vi "Resolve Actions.vi"(7 "Round":u32, 9 "Teams in":refnum<class "Team.lvclass">[](array[class]), 11 "Map in":refnum<class "Map.lvclass">) -> (1 "Teams out":refnum<class "Team.lvclass">[](array[class]), 3 "Map out":refnum<class "Map.lvclass">)   [LabVIEW 2020]
uses:
  Map.lvclass
  0a775b4c-5167-4406-8f15-4eae84d41572.vi
  38daf693-381b-46a9-8c9a-4444c2b0fe34.vi
  ccb221bf-d3dd-4727-afb1-9f97ce610da8.vi
  6b4b9fb7-2456-45d2-a43b-a07e031806e2.vi
  9ad54500-6e5d-40f5-b12a-b38904da31c5.vi
  db824b78-584a-40f1-a452-5d296daad2c0.vi
  ca1b2fc2-8180-4472-9101-8774a23246c0.vi
  Team/Team.lvclass
panel:
  out "Finish":dbl
  out "Attacks":dbl
  out "Replicates":dbl
  out "Moves":dbl
  out "Waits":dbl
  out "Init":dbl
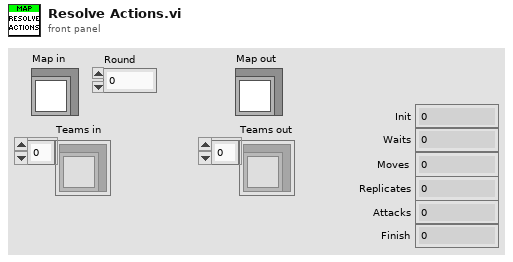
[diagram p1: front panel]
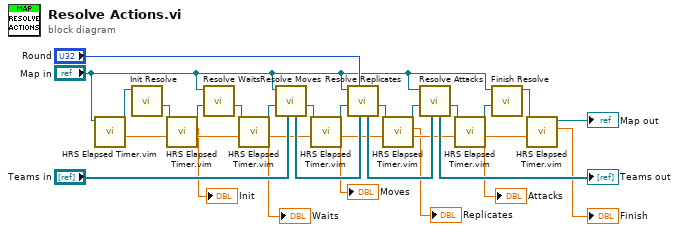
[diagram p0: block diagram]
diagram:
  n1 = call "HRS Elapsed Timer.vim"("Top In"="Map in") -> ("HRS"=w3:dbl, "Top"=w23:refnum<class "Map.lvclass">)  [unwired: 7 in, 2 out]
  n2 = call "Init Resolve.vi"("Map in"=w23) -> ("New Map out"=w26:refnum<class "Map.lvclass">)  [unwired: 10 in]
  n3 = call "HRS Elapsed Timer.vim"("HRS In"=w3, "Top In"=w26) -> ("HRS"=w21:dbl, "Elapsed"=→"Init":dbl, "Top"=w25:refnum<class "Map.lvclass">)  [unwired: 6 in, 1 out]
  n4 = call "Resolve Waits.vi"("New Map in"=w25, "Map in"="Map in") -> ("New Map out"=w10:refnum<class "Map.lvclass">)  [unwired: 9 in]
  n5 = call "HRS Elapsed Timer.vim"("HRS In"=w21, "Top In"=w10) -> ("HRS"=w20:dbl, "Elapsed"=→"Waits":dbl, "Top"=w9:refnum<class "Map.lvclass">)  [unwired: 6 in, 1 out]
  n6 = call "Resolve Moves.vi"("Teams in"="Teams in", "New Map in"=w9, "Map in"="Map in") -> ("New Map out"=w12:refnum<class "Map.lvclass">, "Teams out"=w29:refnum<class "Team.lvclass">[])  [unwired: 7 in]
  n7 = call "HRS Elapsed Timer.vim"("HRS In"=w20, "Top In"=w12) -> ("HRS"=w19:dbl, "Elapsed"=→"Moves":dbl, "Top"=w11:refnum<class "Map.lvclass">)  [unwired: 6 in, 1 out]
  n8 = call "Resolve Replicates.vi"("Teams in"=w29, "Round"="Round", "New Map in"=w11, "Map in"="Map in") -> ("New Map out"=w14:refnum<class "Map.lvclass">, "Teams out"=w28:refnum<class "Team.lvclass">[])  [unwired: 6 in]
  n9 = call "HRS Elapsed Timer.vim"("HRS In"=w19, "Top In"=w14) -> ("HRS"=w18:dbl, "Elapsed"=→"Replicates":dbl, "Top"=w13:refnum<class "Map.lvclass">)  [unwired: 6 in, 1 out]
  n10 = call "Resolve Attacks.vi"("Teams in"=w28, "New Map in"=w13, "Map in"="Map in") -> ("New Map out"=w16:refnum<class "Map.lvclass">, "Teams out"=→"Teams out":refnum<class "Team.lvclass">[])  [unwired: 7 in]
  n11 = call "HRS Elapsed Timer.vim"("HRS In"=w18, "Top In"=w16) -> ("HRS"=w17:dbl, "Elapsed"=→"Attacks":dbl, "Top"=w15:refnum<class "Map.lvclass">)  [unwired: 6 in, 1 out]
  n12 = call "Finish Resolve.vi"("New Map in"=w15, "Map in"="Map in") -> ("Map out"=w22:refnum<class "Map.lvclass">)  [unwired: 9 in]
  n13 = call "HRS Elapsed Timer.vim"("HRS In"=w17, "Top In"=w22) -> ("Elapsed"=→"Finish":dbl, "Top"=→"Map out":refnum<class "Map.lvclass">)  [unwired: 6 in, 2 out]
